vi "CleanUpReply.vi"(11 "String":string) -> (3 "Cleaned string":string)   [LabVIEW 2020]
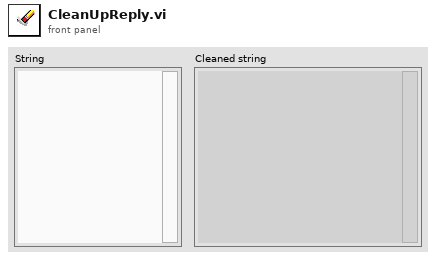
[diagram p1: front panel]
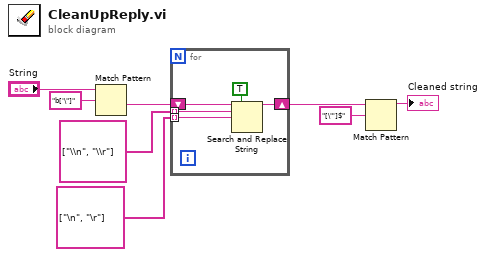
[diagram p0: block diagram]
diagram:
  n1 = Match Pattern(string="String", regular expression="b['\"]") -> (after substring=w5:string)  [unwired: 1 in, 3 out]
  n2 = for {
    shift-right: [w13] -> w7
    shift-left: w5 -> [w11]
    tunnel: string[] ["\\n", "\\r"] -> [w10] mode=indexing
    tunnel: string[] ["\n", "\r"] -> [w9] mode=indexing
    n3 = Search and Replace String(replace all?=TRUE ("replace all? (F)"), input string=w11, search string=w10, replace string=w9) -> (result string=w13:string)  [unwired: 4 in, 3 out]
  }
  n4 = Match Pattern(string=w7, regular expression="[\"']$") -> (before substring=→"Cleaned string":string)  [unwired: 1 in, 3 out]
